vi "20151030 gyro+accel+kalman filter+UL sensor+servo test.vi"() -> ()   [LabVIEW 2013]
uses:
  <vilib>/MakerHub/LINX/Public/Sensors/Accelerometer/MPU60X0/DeviceAddresses.ctl
  <vilib>/MakerHub/LINX/Public/Sensors/Accelerometer/MPU60X0/AccelFullScaleRanges.ctl
  <vilib>/MakerHub/LINX/Public/Sensors/Accelerometer/MPU60X0/GyroFullScaleRanges.ctl
  <vilib>/Analysis/baseanly.llb/Mean (DBL).vi
  <vilib>/MakerHub/LINX/Public/Sensors/Motion/Servo/Servo Open N Channels.vi
  <vilib>/MakerHub/LINX/Public/Sensors/Motion/Servo/Servo Close N Channels.vi
  <vilib>/MakerHub/LINX/Public/Sensors/Motion/Servo/Servo Set Pulse Width N Channels.vi
  <vilib>/addons/Time Series Analysis/Series Preprocess.llb/TSA Moving Average (Array).vi
  <vilib>/MakerHub/LINX/LMH-LINX.lvlib
  <vilib>/MakerHub/LINX/Public/Sensors/Motion/Servo/Servo.lvlib
  <vilib>/MakerHub/LINX/Public/Sensors/Ultrasonic/Ultrasonic.lvlib
  <vilib>/MakerHub/LINX/Public/Sensors/Accelerometer/MPU60X0/MPU60X0.lvlib
  <vilib>/addons/_Advanced Signal Processing/NI_AdvSigProcTSA.lvlib
  <vilib>/Analysis/NI_AALBase.lvlib
panel:
  in  "Initial Pulse Widths (uS) 3":u16[](array[numeric])=[1100, 900, 2100, 1500, 1500, 600, 1600, 2100, 600, 1400, 700, 600] min=600 max=2400 step=100
  out "Waveform Chart":cluster{"x_angle":dbl, "x_angle":dbl}(graph)={"x_angle"=1.9931978450377157, "x_angle"=-3.785425420621641}
  in  "Moving avg?":bool=TRUE
  out "After Kalman filter":T1(graph)={"pitch"=2.1263282656039806, "roll"=-2.9456456798246218, "x_angle"=2.1950457671940673, "x_angle"=-3.587569186059353}
  out "roll":dbl=-3.587569186059353
  out "pitch":dbl=2.1950457671940673
  out "Error Out":errorcluster
  in  "Servo Channels":u8[](array[numeric])=[2, 3, 4, 5, 6, 7, 8, 9, 10, 11, 12, 13]
  in  "error in (no error)":errorcluster
  out "Initialize OK?":bool=TRUE
  in  "Stop Button":bool
  in  "Serial Port":refnum<visa-resource-name>="COM10"
  # "up: CK"
  # "up: CK"
  # "up: CCK"
  # "up: CK"
  # "up: CK"
  # "up: CCK"
  # "up: CK"
  # "up: CK"
  # "up: CCK"
  # "up: CK"
  # "up: CK"
  # "up: CCK"
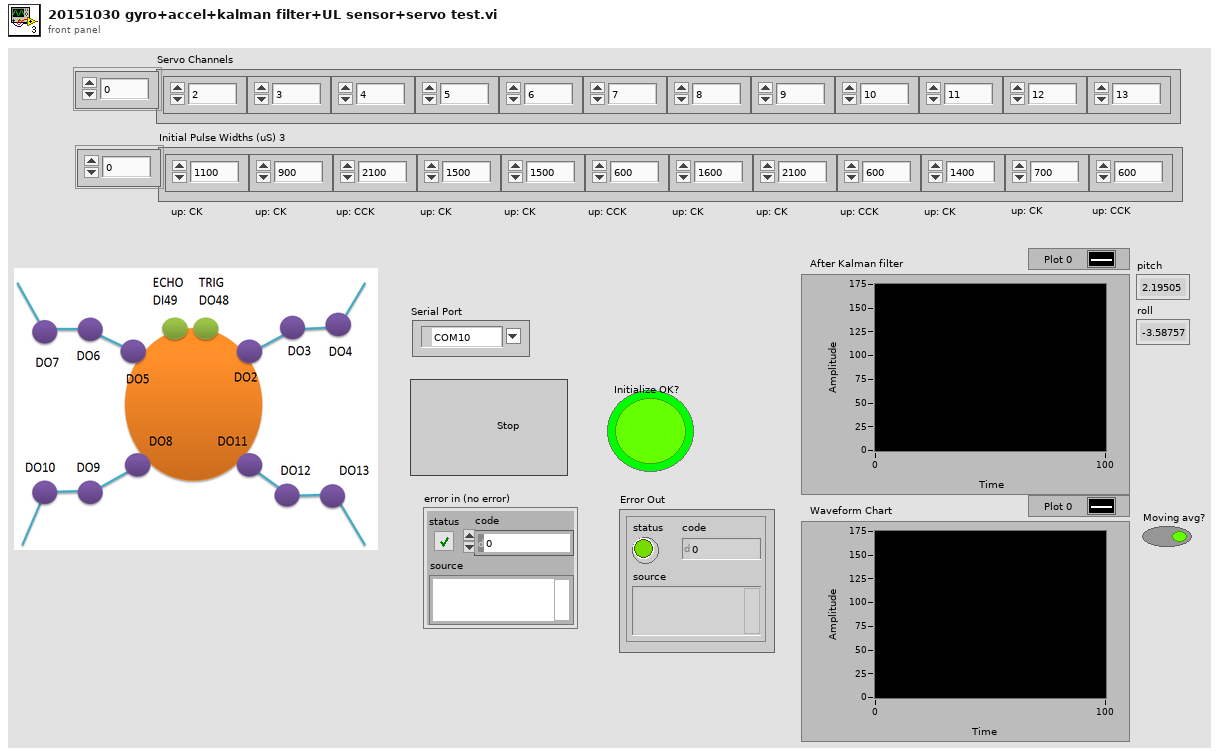
[diagram p1: front panel]
types:
  T1 = cluster{"pitch":dbl, "roll":dbl, "x_angle":dbl, "x_angle":dbl}
  T2 = typedef "LMH-LINX.lvlib/MPU60X0.lvlib/GyroFullScaleRanges.ctl" = enum8{"±250 °/s", "±500 °/s", "±1000 °/s", "±2000 °/s"}
  T3 = typedef "LMH-LINX.lvlib/MPU60X0.lvlib/AccelFullScaleRanges.ctl" = enum16{"±2g", "±4g", "±8g", "±16g"}
  T4 = typedef "LMH-LINX.lvlib/MPU60X0.lvlib/DeviceAddresses.ctl" = enum16{"0x68", "0x69"}
  T5 = typedef "LMH-LINX.lvlib/LINX Ref.ctl" = cluster{"Platform":T6, "Interface":T7, "LINX Device Config":T8}
  T6 = typedef "LMH-LINX.lvlib/Platform.ctl" = enum16{"LINX", "myRIO"}
  T7 = typedef "LMH-LINX.lvlib/Interface.ctl" = enum16{"Serial", "TCP"}
  T8 = typedef "LMH-LINX.lvlib/Device.lvlib/LINX Device Config.ctl" = cluster{"Interface":T7, "COM Port":refnum<visa-resource-name>, "TCP Configuration":T9, "Device Family":u8, "Device ID":u8, "Device Name":string, "TCP Ref":refnum<k5>, "Channels":T10}
  T9 = typedef "LMH-LINX.lvlib/Device.lvlib/TCP Config.ctl" = cluster{"IP Address":string, "Port":u16}
  T10 = typedef "LMH-LINX.lvlib/Channels.ctl" = cluster{"DI":u8[], "DO":u8[], "AI":u8[], "AO":u8[], "PWM":u8[], "QE":u8[], "UART":u8[], "I2C 2":u8[], "SPI":u8[], "CAN":u8[], "Servo":u8[], "AI Ref (V)":dbl, "AO Ref (V)":dbl, "AO Resolution (Bits)":u8}
  T11 = cluster{"X Axis":i16, "Y Axis":i16, "Z Axis":i16}
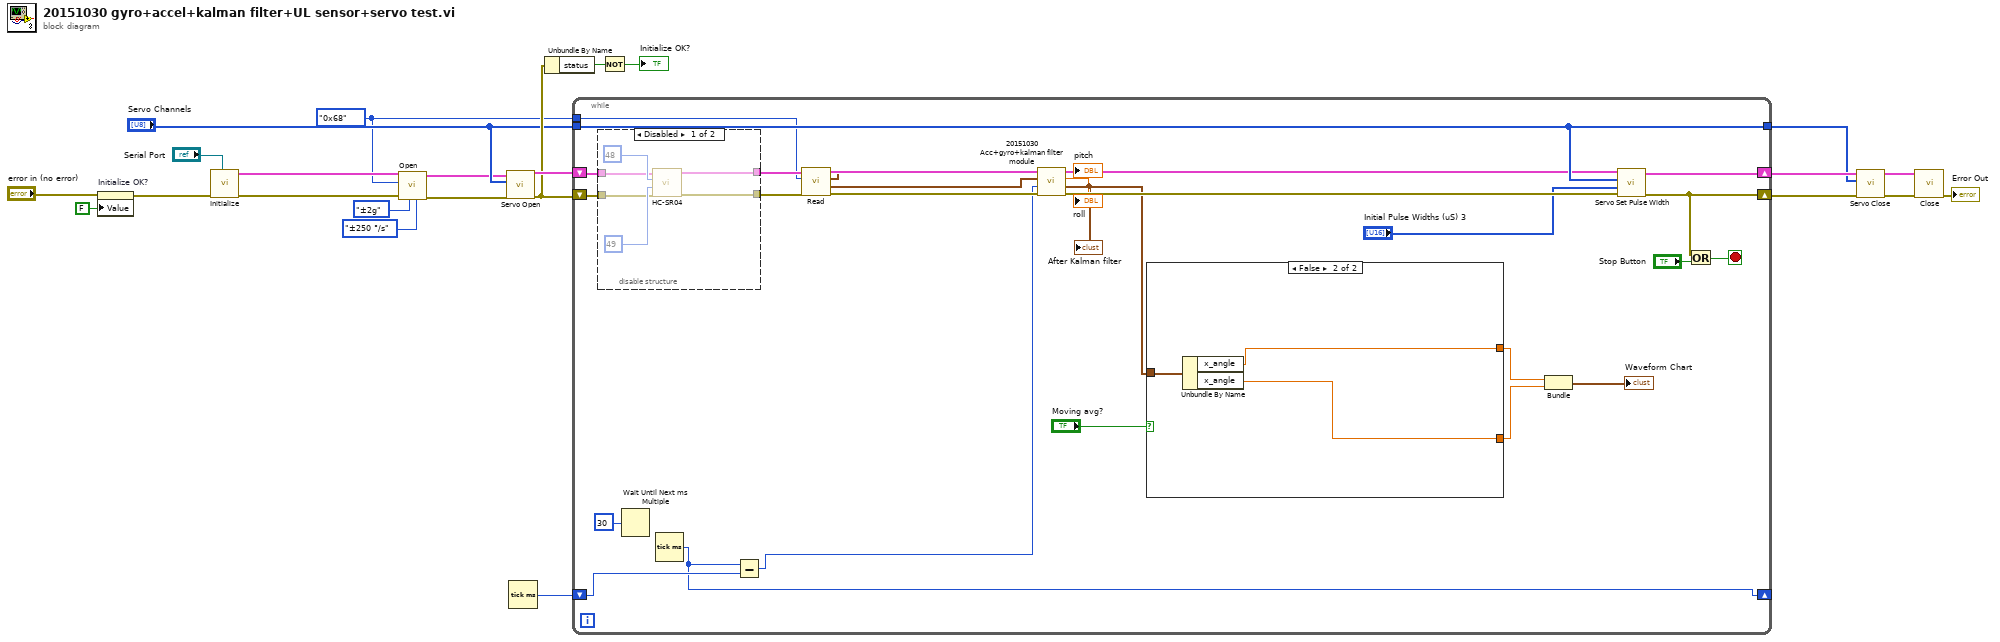
[diagram p0: block diagram]
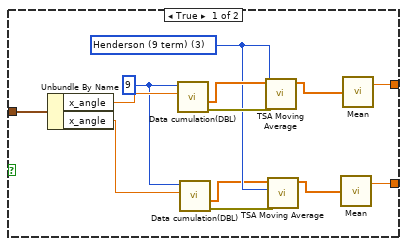
[diagram p2: hidden frame]
diagram:
  w5 = DeviceAddresses."0x68" ("Device Address")
  n1 = property on="Initialize OK?" class="Bool (strict)"(error in="error in (no error)", "Value"=FALSE ("Initialize OK?")) -> (error out=w14:errorcluster)  [unwired: 1 in, 1 out]
  n2 = call <vilib>:"Initialize.vi"("Serial Port"="Serial Port", "Error In"=w14) -> ("Error Out"=w8:errorcluster, "LINX Ref"=w9:T5)  [unwired: 7 in, 1 out]
  n3 = call <vilib>:"Open.vi"("Gyro Full Scale Range"=GyroFullScaleRanges."±250 °/s", "Accel Full Scale Range"=AccelFullScaleRanges."±2g", "Error In"=w8, "Device Address"=w5, "LINX Resource"=w9) -> ("Error Out"=w6:errorcluster, "LINX Resource"=w7:T5)  [unwired: 5 in]
  n4 = call-poly <vilib>:"Servo Open.vi"("Error In"=w6, "Servo Channels"="Servo Channels", "LINX Resource"=w7) -> ("Error Out"=w17:errorcluster, "LINX Resource"=w22:T5)  [unwired: 7 in]
  n5 = Tick Count (ms)() -> (millisecond timer value=w1:u32)
  n6 = Unbundle By Name(w17) -> ("status"=w16:bool)
  n7 = while {
    shift-right: [w48] -> w18
    shift-left: w17 -> [w44]
    tunnel: "Servo Channels" -> [w46]
    shift-right: [w47] -> w21
    shift-left: w22 -> [w45]
    tunnel: [w46] -> w10
    tunnel: w5 -> [w39]
    shift-right: [w30] -> _
    shift-left: w1 -> [w34]
    stop <- w50 stop-if-true
    n8 = disable-structure shown="Disabled" {
      disable-tunnel: w45 -> [w70 w74]
      disable-tunnel: w44 -> [w69 w73]
      disable-tunnel: [w68 w73] -> w42
      disable-tunnel: [w67 w74] -> w41
      frame Disabled {
        n9 = call <vilib>:"HC-SR04.vi"("Error In"=w69, "Echo Pin (DI)"=u8 49, "Trig"=u8 48, "LINX Resource"=w70) -> ("Error Out"=w68:errorcluster, "LINX Resource"=w67:T5)  [unwired: 4 in, 2 out]
      }
      frame Enabled {
      }
    }
    n10 = Wait Until Next ms Multiple(millisecond multiple=u32 30) -> ()  [unwired: 1 out]
    n11 = Tick Count (ms)() -> (millisecond timer value=w30:u32)
    n12 = Subtract(x=w30, y=w34) -> (x-y=w33:u32)
    n13 = call <vilib>:"Read.vi"("Error In"=w42, "Device Address"=w39, "LINX Resource"=w41) -> ("Error Out"=w36:errorcluster, "Gyro  Data"=w37:T11, "Acceleration Data"=w38:T11, "LINX Resource"=w40:T5)  [unwired: 4 in, 1 out]
    n14 = call "20151030 Acc+gyro+kalman filter module.vi"("error in (no error)"=w36, "Looptime"=w33, "Gyro  Data"=w37, "Acceleration Data"=w38) -> ("error out"=w35:errorcluster, "After Kalman filter"=w28:T1, "roll"=→"roll":dbl, "pitch"=→"pitch":dbl)  [unwired: 4 in]
    "After Kalman filter" <- w28
    n15 = case shown="False" "Moving avg?" {
      tunnel: w28 -> [w63 w66]
      tunnel: [w52 w65] -> w27
      tunnel: [w51 w64] -> w26
      frame True {
        w56 = 3 items=["Spencer (15 term)"=1, "Henderson (7 term)"=2, "Henderson (9 term)"=3, "Henderson (13 term)"=4, "Henderson (23 term)"=5] ("method")
        w57 = 9 ("Sample length")
        n16 = Unbundle By Name(w63) -> ("x_angle"=w62:dbl, "x_angle"=w58:dbl)
        n17 = call "Data cumulation(DBL).vi"("Data in"=w62, "Sample length"=w57) -> ("error out"=w60:errorcluster, "Data out"=w61:dbl[])  [unwired: 6 in, 2 out]
        n18 = call "Data cumulation(DBL).vi"("Data in"=w58, "Sample length"=w57) -> ("error out"=w59:errorcluster, "Data out"=w55:dbl[])  [unwired: 6 in, 2 out]
        n19 = call-poly <vilib>:"TSA Moving Average.vi"("error in (no error)"=w60, "method"=w56, "Xt"=w61) -> ("Xt out"=w54:dbl[])  [unwired: 7 in, 1 out]
        n20 = call-poly <vilib>:"TSA Moving Average.vi"("error in (no error)"=w59, "method"=w56, "Xt"=w55) -> ("Xt out"=w53:dbl[])  [unwired: 7 in, 1 out]
        n21 = call-poly <vilib>:"Mean.vi"("X"=w53) -> ("mean"=w51:dbl)  [unwired: 1 out]
        n22 = call-poly <vilib>:"Mean.vi"("X"=w54) -> ("mean"=w52:dbl)  [unwired: 1 out]
      }
      frame False {
        n23 = Unbundle By Name(w66) -> ("x_angle"=w65:dbl, "x_angle"=w64:dbl)
      }
    }
    n24 = Bundle("x_angle"=w27, "x_angle"=w26) -> (→"Waveform Chart":cluster{"x_angle":dbl, "x_angle":dbl})  [unwired: 1 in]
    n25 = call-poly <vilib>:"Servo Set Pulse Width.vi"("Error In"=w35, "Pulse Widths (uS)"="Initial Pulse Widths (uS) 3", "Servo Channels"=w46, "LINX Resource"=w40) -> ("Error Out"=w48:errorcluster, "LINX Resource"=w47:T5)  [unwired: 6 in]
    n26 = Or(x=w48, y="Stop Button") -> (x .or. y?=w50:bool)
  }
  n27 = Not(x=w16) -> (.not. x?=→"Initialize OK?":bool)
  n28 = call-poly <vilib>:"Servo Close.vi"("Error In"=w18, "Servo Channels"=w10, "LINX Resource"=w21) -> ("Error Out"=w19:errorcluster, "LINX Resource"=w20:T5)  [unwired: 7 in]
  n29 = call <vilib>:"Close.vi"("Error In"=w19, "LINX Resource"=w20) -> ("Error Out"=→"Error Out":errorcluster)  [unwired: 8 in, 1 out]
